vi "MainData.vi"() -> ()   [LabVIEW 2020]
panel:
  in  "Max voltage:":dbl=30.0 min=5.0 format="%#.3gV"
  in  "BufferTime(s)":dbl=2.0 caption="Buffer:" format="%#.3gs"
  in  "ExecuteTime(s)":dbl=5.0 caption="Execute:" min=1.0 format="%#.3gs"
  in  "Step voltage:":dbl=0.1 format="%#.3gV"
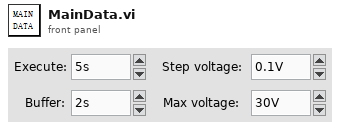
[diagram p1: front panel]
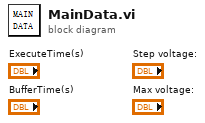
[diagram p0: block diagram]
diagram:
